vi "Update Load State Data.vi"(8 "error in (no error)":errorcluster, 11 "QControl Creation in":refnum<class "QControl Creation.lvclass">) -> (0 "error out":errorcluster, 3 "QControl Creation (dup)":refnum<class "QControl Creation.lvclass">)   [LabVIEW 2015, in "QControl Creation.lvclass"]
doc: "<b> </b> <b> </b>\n©2016 Q Software Innovations, LLC (QSI)\nwritten by Quentin Alldredge\nproduced in LabVIEW 2015\n\nsupport@qsoftwareinnovations.com\nwww.qsoftwareinnovations.com\n\nAll rights reserved.\n\nRedistribution and use in source and binary forms, with or without modification, are permitted provided that the following conditions are met:\n\n * Redistributions of source code must retain the above copyright notice, this list of conditions and the following disclaimer.\n * Redistributions in binary form must reproduce the above copyright notice, this list of conditions and the following disclaimer in the documentation and/or other materials provided with the distribution.\n * Neither the name of Q Software Innovations, LLC. nor the names of its contributors may be used to endorse or promote products derived from this software without specific prior written permission.\n\nTHIS SOFTWARE IS PROVIDED BY THE COPYRIGHT HOLDERS AND CONTRIBUTORS \"AS IS\" AND ANY EXPRESS OR IMPLIED WARRANTIES, INCLUDING, BUT NOT LIMITED TO, THE IMPLIED WARRANTIES OF MERCHANTABILITY AND FITNESS FOR A PARTICULAR PURPOSE ARE DISCLAIMED. IN NO EVENT SHALL THE COPYRIGHT OWNER OR CONTRIBUTORS BE LIABLE FOR ANY DIRECT, INDIRECT, INCIDENTAL, SPECIAL, EXEMPLARY, OR CONSEQUENTIAL DAMAGES (INCLUDING, BUT NOT LIMITED TO, PROCUREMENT OF SUBSTITUTE GOODS OR SERVICES; LOSS OF USE, DATA, OR PROFITS; OR BUSINESS INTERRUPTION) HOWEVER CAUSED AND ON ANY THEORY OF LIABILITY, WHETHER IN CONTRACT, STRICT LIABILITY, OR TORT (INCLUDING NEGLIGENCE OR OTHERWISE) ARISING IN ANY WAY OUT OF THE USE OF THIS SOFTWARE, EVEN IF ADVISED OF THE POSSIBILITY OF SUCH DAMAGE."
uses:
  QControl Creation.lvclass
  QControl Creation.lvclass/QControl Creation.ctl
  <vilib>/Utility/traverseref.llb/TRef TravTarget.ctl
  <vilib>/Utility/error.llb/Error Cluster From Error Code.vi
  <vilib>/ErrorRing/Error Ring.xnode
  <vilib>/Utility/traverseref.llb/VI Scripting - Traverse.lvlib
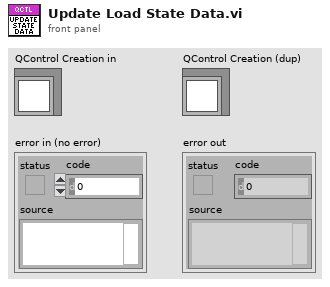
[diagram p1: front panel]
types:
  T1 = typedef "TRef TravTarget.ctl" = enum16{"FP", "BD", "Other"}
  T2 = typedef "LVPositionTypeDef.ctl" = cluster{"Left":i32, "Top":i32}
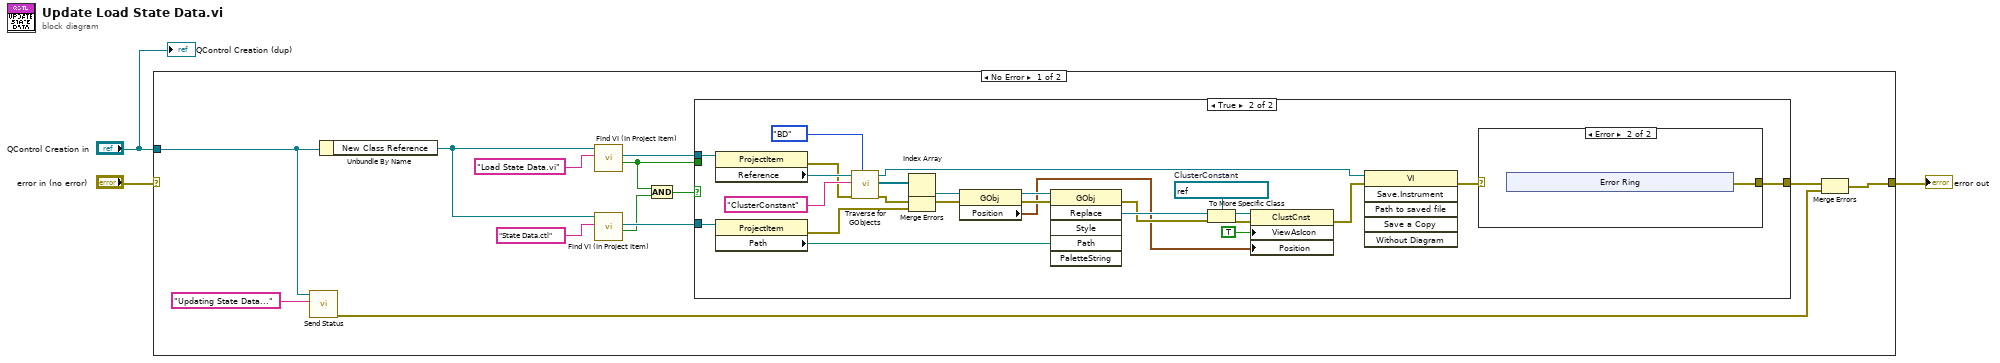
[diagram p0: block diagram]
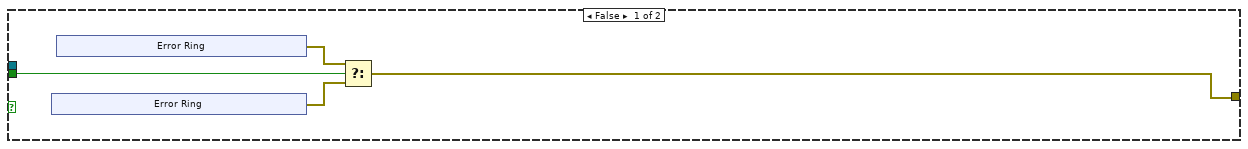
[diagram p2: hidden frame]
diagram:
  n1 = case shown="No Error" "error in (no error)" {
    selector: "error in (no error)" -> [_ w63]
    tunnel: [w5 w63] -> w2
    tunnel: "QControl Creation in" -> [w9 _]
    frame No Error {
      n2 = call "Send Status.vi"("Status"="Updating State Data..." ("Add Item"), "QControl Creation in"=w9) -> ("error out (dup)"=w4:errorcluster)  [unwired: 8 in, 1 out]
      n3 = Unbundle By Name(w9) -> ("New Class Reference"=w13:refnum<vi>)
      n4 = call "Find VI (In Project Item).vi"("VI Name"="Load State Data.vi", "ProjectItem in"=w13) -> ("Found?"=w6:bool, "VI ProjectItem Refnum"=w15:refnum<vi>)  [unwired: 7 in, 1 out]
      n5 = call "Find VI (In Project Item).vi"("VI Name"="State Data.ctl", "ProjectItem in"=w13) -> ("Found?"=w8:bool, "VI ProjectItem Refnum"=w12:refnum<vi>)  [unwired: 7 in, 1 out]
      n6 = And(x=w6, y=w8) -> (x .and. y?=w7:bool)
      n7 = case shown="True" w7 {
        tunnel: w15 -> [_ w55]
        tunnel: w12 -> [_ w48]
        tunnel: [w17 w31] -> w11
        tunnel: w6 -> [w20 _]
        frame False {
          n8 = xnode "Error Ring"() -> ("error out"=w19:errorcluster)
          n9 = xnode "Error Ring"() -> ("error out"=w18:errorcluster)
          n10 = Select(t=w18, s=w20, f=w19) -> (s? t:f=w17:errorcluster)
        }
        frame True {
          w39 = refnum<vi> refnum  # ClusterConstant
          n11 = property class="ProjectItem"(reference=w55) -> (error out=w51:errorcluster, "Reference"=w54:refnum<vi>)  [unwired: 1 in, 1 out]
          n12 = property class="ProjectItem"(reference=w48) -> (error out=w46:errorcluster, "Path"=w47:path)  [unwired: 1 in, 1 out]
          n13 = call <vilib>:"Traverse for GObjects.vi"("Traverse Target"=TRef_TravTarget."BD", "error in (no error)"=w51, "Class Name"="ClusterConstant", "VI Refnum"=w54) -> ("error out"=w49:errorcluster, "References"=w50:refnum<vi>[], "dup VI Refnum"=w44:refnum<vi>)  [unwired: 4 in, 1 out]
          n14 = Index Array(array=w50) -> (element=w41:refnum<vi>)  [unwired: 1 in]
          n15 = Merge Errors(w49, w46) -> (w45:errorcluster)
          n16 = property class="GObj"(reference=w41, error in=w45) -> (reference out=w40:refnum<vi>, error out=w42:errorcluster, "Position"=w33:T2)
          n17 = invoke class="GObj" method="Replace"(reference=w40, error in=w42, "Path"=w47) -> (error out=w38:errorcluster, "Replace"=w43:refnum<vi>)  [unwired: 3 in, 4 out]
          n18 = To More Specific Class(target class=w39, reference=w43, error in=w38) -> (specific class reference=w37:refnum<vi>, error out=w36:errorcluster)
          n19 = property class="ClustCnst"(reference=w37, error in=w36, "ViewAsIcon"=TRUE ("View As Icon"), "Position"=w33) -> (error out=w34:errorcluster)  [unwired: 1 out]
          n20 = invoke class="VI" method="Save.Instrument"(reference=w44, error in=w34) -> (error out=w32:errorcluster)  [unwired: 4 in, 5 out]
          n21 = case shown="Error" w32 {
            selector: w32 -> [w56 _]
            tunnel: [w56 w57] -> w31
            frame No Error {
            }
            frame Error {
              n22 = xnode "Error Ring"() -> ("error out"=w57:errorcluster)
            }
          }
        }
      }
      n23 = Merge Errors(w11, w4) -> (w5:errorcluster)
    }
    frame Error {
    }
  }
  "error out" <- w2
  "QControl Creation (dup)" <- "QControl Creation in"
